vi "CLD 5 Parse Config Data File.vi"(8 "error in (no error)":errorcluster, 10 "Array In":T1[][](array[typedef])=[[{"Numeric"=1.25, "Boolean"=FALSE, "String"="One"}, {"Numeric"=1.35, "Boolean"=TRUE, "String"="Two"}, {"Numeric"=1.5, "Boolean"=FALSE, "String"="Three"}, {"Numeric"=1.0, "Boolean"=TRUE, "String"="Four"}], [{"Numeric"=2.0, "Boolean"=TRUE, "String"="Five"}, {"Numeric"=0.75, "Boolean"=FALSE, "String"="Six"}, {"Numeric"=0.9, "Boolean"=TRUE, "String"="Seven"}, {"Numeric"=0.75, "Boolean"=FALSE, "String"="Eight"}]], 11 "Get/Set":enum16{"Get", "Set"}(ring)) -> (0 "error out":errorcluster, 3 "Array Out":T1[][](array[typedef]))   [LabVIEW 2019]
doc: "CLD 5 exercise"
uses:
  CLD 5 Data Cluster.ctl
  <vilib>/Utility/config.llb/Write Key (Double).vi
  <vilib>/Utility/config.llb/Write Key (Boolean).vi
  <vilib>/Utility/config.llb/Write Key (String).vi
  <vilib>/Utility/config.llb/NI_LVConfig.lvlib
panel:
  out "Array":T1
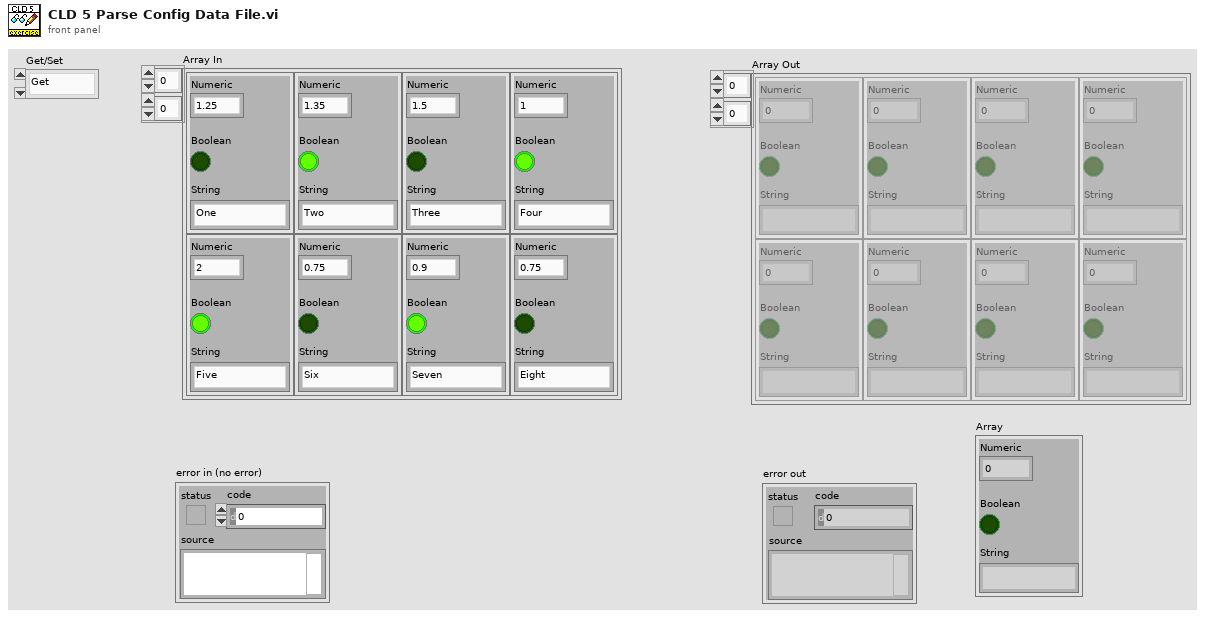
[diagram p1: front panel]
types:
  T1 = typedef "CLD 5 Data Cluster.ctl" = cluster{"Numeric":dbl, "Boolean":bool, "String":string}
  T2 = typedef "NI_LVConfig.lvlib/Config Data RefNum.ctl" = refnum<k1>
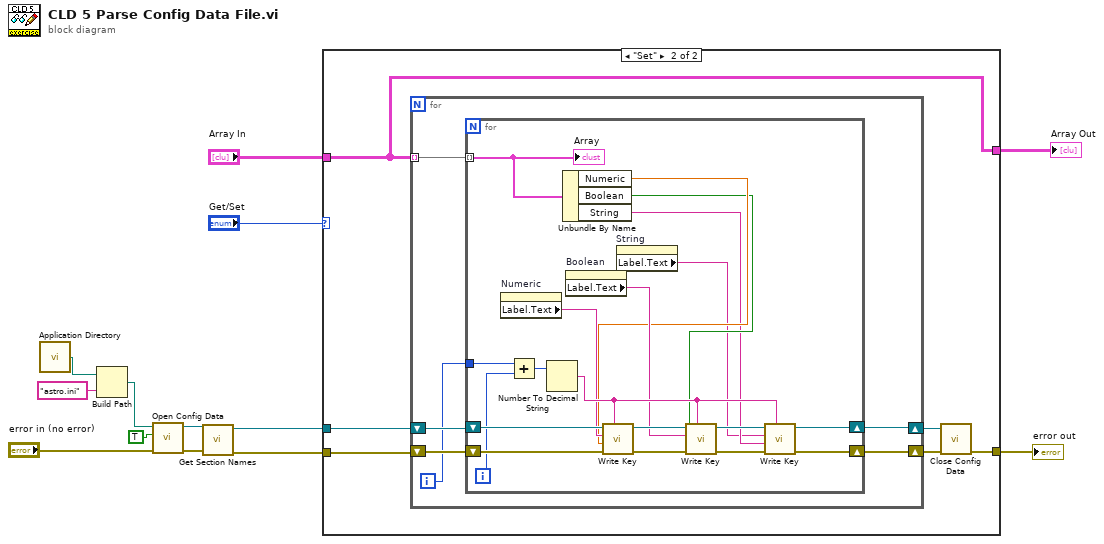
[diagram p0: block diagram]
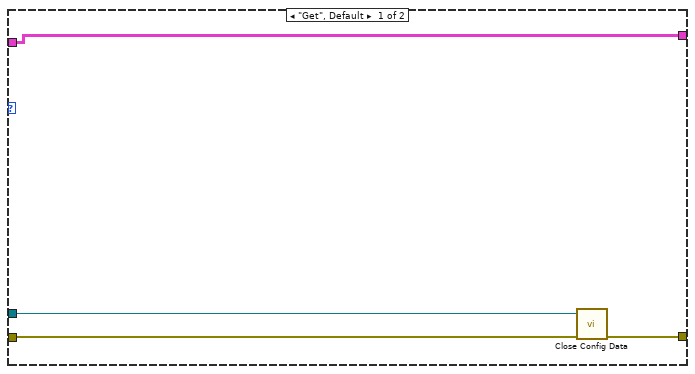
[diagram p2: hidden frame]
diagram:
  n1 = call <vilib>:"Application Directory.vi"() -> ("Application Directory"=w12:path)
  n2 = Build Path(base path=w12, name or relative path="astro.ini") -> (appended path=w10:path)
  n3 = call <vilib>:"Open Config Data.vi"("error in (no error)"="error in (no error)", "create file if necessary (T)"=TRUE, "configuration file path"=w10) -> ("error out"=w8:errorcluster, "refnum"=w7:T2)  [unwired: 6 in, 1 out]
  n4 = call <vilib>:"Get Section Names.vi"("error in (no error)"=w8, "refnum"=w7) -> ("error out"=w5:errorcluster, "refnum out"=w4:T2)  [unwired: 7 in, 1 out]
  n5 = case shown="\"Set\"" "Get/Set" {
    tunnel: w5 -> [w15 w23]
    tunnel: w4 -> [w14 w21]
    tunnel: [w16 w19] -> w1
    tunnel: "Array In" -> [w17 w22]
    tunnel: [w17 w22] -> w2
    frame "Get", Default {
      n6 = call <vilib>:"Close Config Data.vi"("error in (no error)"=w15, "refnum"=w14) -> ("error out"=w16:errorcluster)  [unwired: 8 in, 1 out]
    }
    frame "Set" {
      n7 = for {
        shift-right: [w27] -> w20
        shift-left: w23 -> [w28]
        tunnel: w22 -> [w29] mode=indexing
        shift-right: [w25] -> w18
        shift-left: w21 -> [w26]
        i -> [w24]
        n8 = for {
          tunnel: w29 -> [w46] mode=indexing
          shift-right: [w38] -> w27
          shift-left: w28 -> [w48]
          shift-right: [w37] -> w25
          shift-left: w26 -> [w47]
          tunnel: w24 -> [w45]
          i -> [w44]
          n9 = property on="Numeric" class="DigNum (strict)"() -> ("Label.Text"=w35:string)  [unwired: 2 in, 2 out]
          n10 = Add(x=w45, y=w44) -> (x+y=w43:i32)
          n11 = Number To Decimal String(number=w43) -> (decimal integer string=w36:string)  [unwired: 1 in]
          n12 = Unbundle By Name(w46) -> ("Numeric"=w33:dbl, "Boolean"=w32:bool, "String"=w31:string)
          n13 = property on="Boolean" class="Bool (strict)"() -> ("Label.Text"=w34:string)  [unwired: 2 in, 2 out]
          n14 = call-poly <vilib>:"Write Key.vi"("section"=w36, "error in (no error)"=w48, "value"=w33, "key"=w35, "refnum"=w47) -> ("error out"=w42:errorcluster, "refnum out"=w41:T2)  [unwired: 4 in, 1 out]
          n15 = property on="String" class="Str"() -> ("Label.Text"=w30:string)  [unwired: 2 in, 2 out]
          n16 = call-poly <vilib>:"Write Key.vi"("section"=w36, "error in (no error)"=w42, "value"=w32, "key"=w34, "refnum"=w41) -> ("error out"=w39:errorcluster, "refnum out"=w40:T2)  [unwired: 4 in, 1 out]
          n17 = call-poly <vilib>:"Write Key.vi"("section"=w36, "error in (no error)"=w39, "value"=w31, "key"=w30, "refnum"=w40) -> ("error out"=w38:errorcluster, "refnum out"=w37:T2)  [unwired: 4 in, 1 out]
          "Array" <- w46
        }
      }
      n18 = call <vilib>:"Close Config Data.vi"("error in (no error)"=w20, "refnum"=w18) -> ("error out"=w19:errorcluster)  [unwired: 8 in, 1 out]
    }
  }
  "error out" <- w1
  "Array Out" <- w2
